vi "GetData.vi"() -> ()   [LabVIEW 2011]
uses:
  <vilib>/Platform/TimedLoop/XDataNode/timing_clust.ctl
  <vilib>/Platform/TimedLoop/XDataNode/nitl_modes.ctl
  <vilib>/Platform/TimedLoop/XDataNode/wakeup.ctl
  GlobalVariables.vi
  DS/DSRead int16.vi
  DS/DSRead uint8.vi
  DS/DSRead uint32.vi
  <vilib>/Platform/TimedLoop/XDataNode/XDataNode.xnode
  <vilib>/Platform/TimedLoop/XDataNode/XDNodeRunTimeDep.lvlib
  DS/DSWrite uint32.vi
panel:
  in  "Reinitialize?":bool
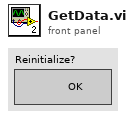
[diagram p1: front panel]
types:
  T1 = enum16{"Read", "Write", "ReadWrite", "BufferedRead", "BufferedReadWrite"}
  T2 = enum16{"OPC Server", "Global", "Dnet1", "Dnet2", "Dnet3", "Ain1", "Ain2", "Aout1", "Din1", "Din2", "Dout1"}
  T3 = typedef "XDNodeRunTimeDep.lvlib/timing_clust.ctl" = cluster{"Expected End [f-1]":u64, "Actual End [f-1]":u64, "Finished Late? [f-1]":bool, "Expected End [i-1]":u64, "Actual End [i-1]":u64, "Finished Late? [i-1]":bool, "Expected Start [i]":u64, "Actual Start [i]":u64, "Expected Start [f]":u64, "Actual Start [f]":u64, "Source Name":string, "Structure Name":string, "Period":i64, "Deadline":i64, "Offset":i64, "Start":i64, "Priority":i32, "Timeout":i32, "Mode":T4, "Wakeup Reason":T5, "Error":errorcluster, "Source Type":string, "Secondary Source Type":string, "Global End Time":u64, "Global Start Time":u64, "Frame Duration":u64, "Iteration Duration":u64, "Assigned CPU":i32, "I/O Scan Engine Mode":u32}
  T4 = typedef "XDNodeRunTimeDep.lvlib/nitl_modes.ctl" = enum32{"No Change", "Process missed periods, maintain original phase", "Discard missed periods, maintain original phase", "Process missed periods, ignore original phase", "Discard missed periods, ignore original phase"}
  T5 = typedef "XDNodeRunTimeDep.lvlib/wakeup.ctl" = enum32{"Normal", "Aborted", "Asynchronous wakeup", "Timing source error", "Timed loop error", "Timeout"}
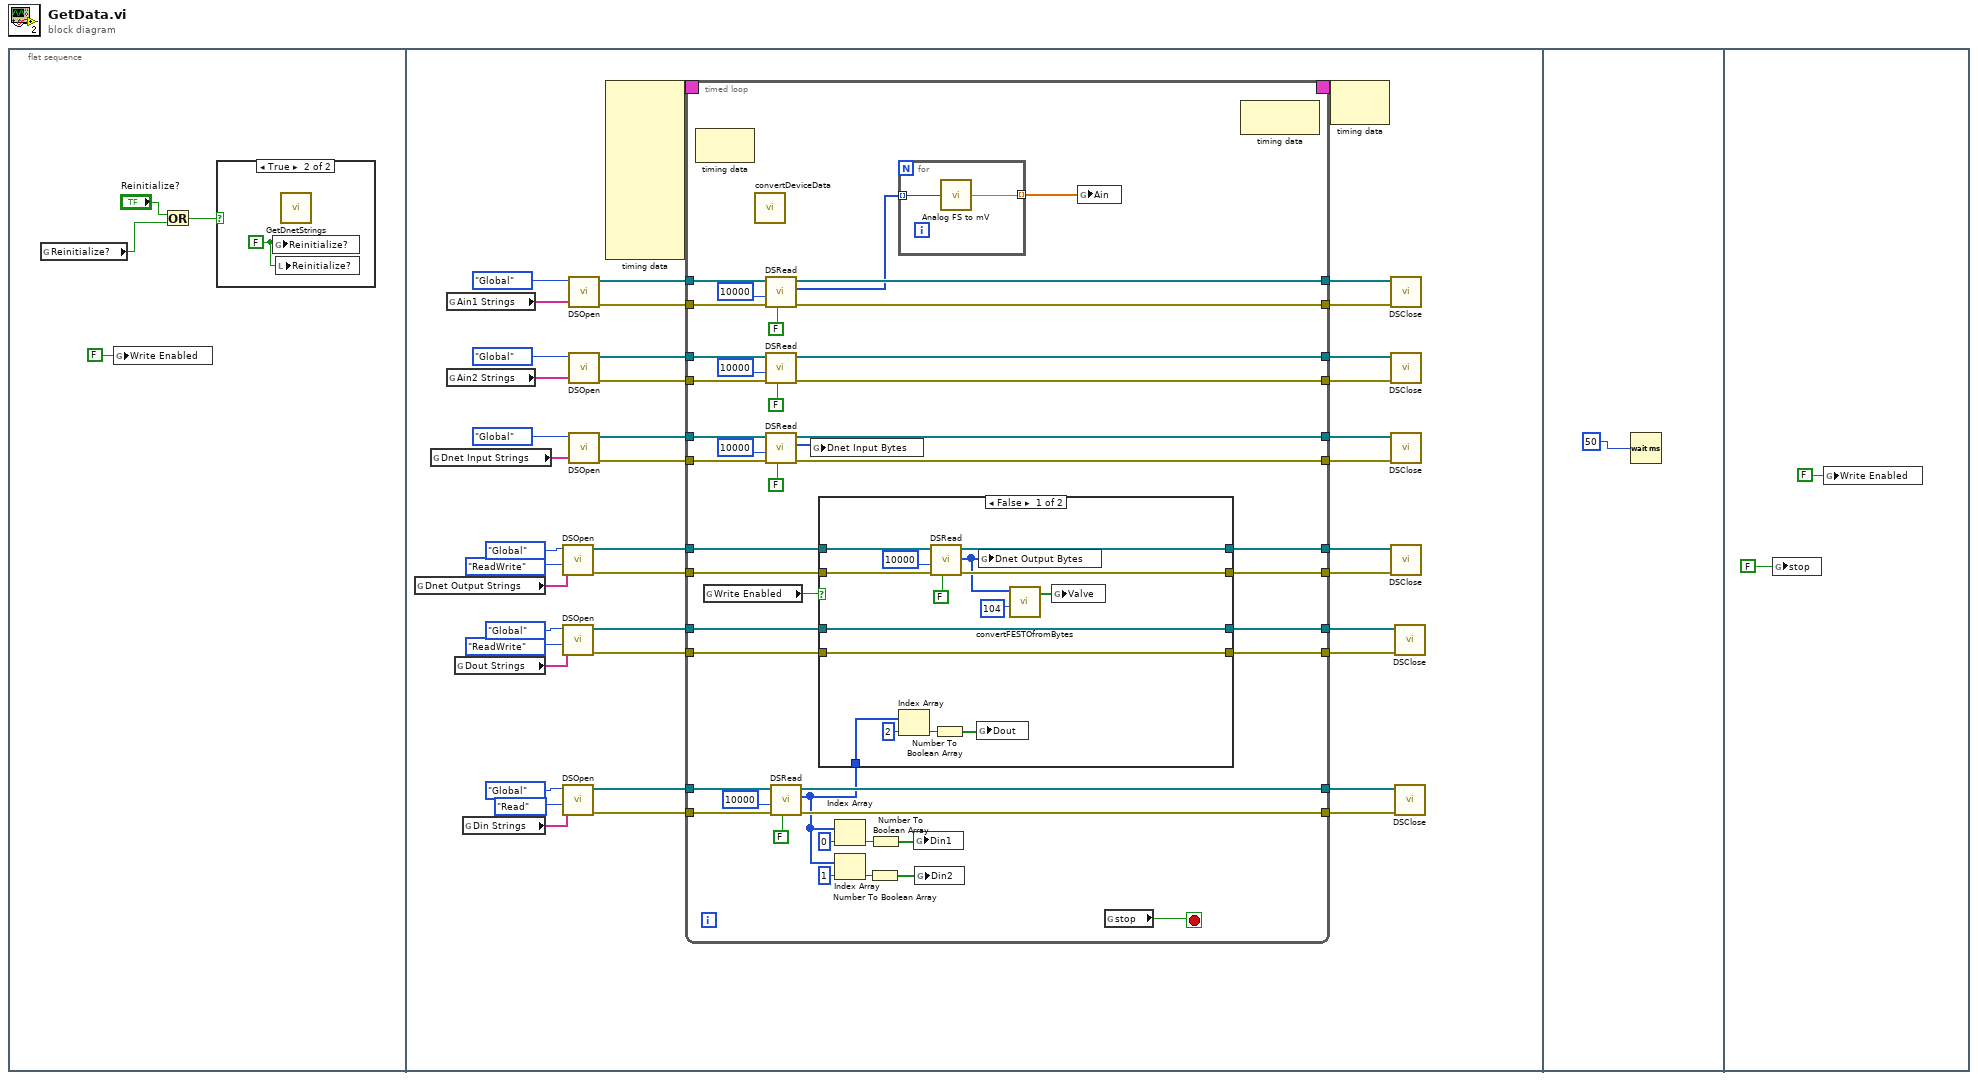
[diagram p0: block diagram]
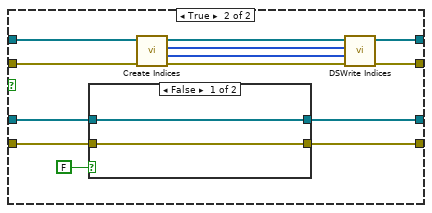
[diagram p3: hidden frame]
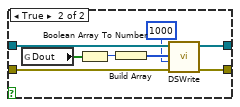
[diagram p4: hidden frame]
diagram:
  n1 = flat-sequence {
    frame #0 {
      n2 = global read "GlobalVariables.vi" "Reinitialize?"() -> (w3:bool)
      n3 = global write "GlobalVariables.vi" "Write Enabled"(FALSE ("Reinitialize?")) -> ()
      n4 = Or(x="Reinitialize?", y=w3) -> (x .or. y?=w2:bool)
      n5 = case shown="True" w2 {
        frame False {
        }
        frame True {
          w5 = FALSE
          n6 = global write "GlobalVariables.vi" "Reinitialize?"(w5) -> ()
          n7 = local write "Reinitialize?"(w5) -> ()
          n8 = call "GetDnetStrings.vi"() -> ()  [unwired: 12 in]
        }
      }
    }
    frame #1 {
      n9 = global read "GlobalVariables.vi" "Dnet Output Strings"() -> (w25:string[])
      n10 = global read "GlobalVariables.vi" "Dnet Input Strings"() -> (w31:string[])
      n11 = global read "GlobalVariables.vi" "Ain1 Strings"() -> (w43:string[])
      n12 = global read "GlobalVariables.vi" "Ain2 Strings"() -> (w37:string[])
      n13 = global read "GlobalVariables.vi" "Dout Strings"() -> (w11:string[])
      n14 = global read "GlobalVariables.vi" "Din Strings"() -> (w18:string[])
      n15 = call "DSOpen.vi"("Array"=w25, "mode"=T1."ReadWrite", "Slot"=T2."Global") -> ("error Out"=w23:errorcluster[], "connection out"=w22:refnum<k13>[])  [unwired: 7 in]
      n16 = call "DSOpen.vi"("Array"=w11, "mode"=T1."ReadWrite", "Slot"=T2."Global") -> ("error Out"=w9:errorcluster[], "connection out"=w8:refnum<k13>[])  [unwired: 7 in]
      n17 = call "DSOpen.vi"("Array"=w18, "mode"=T1."Read", "Slot"=T2."Global") -> ("error Out"=w16:errorcluster[], "connection out"=w15:refnum<k13>[])  [unwired: 7 in]
      n18 = call "DSOpen.vi"("Array"=w43, "Slot"=T2."Global") -> ("error Out"=w42:errorcluster[], "connection out"=w41:refnum<k13>[])  [unwired: 8 in]
      n19 = call "DSOpen.vi"("Array"=w37, "Slot"=T2."Global") -> ("error Out"=w36:errorcluster[], "connection out"=w35:refnum<k13>[])  [unwired: 8 in]
      n20 = call "DSOpen.vi"("Array"=w31, "Slot"=T2."Global") -> ("error Out"=w29:errorcluster[], "connection out"=w30:refnum<k13>[])  [unwired: 8 in]
      n21 = node-c288() -> (w46:T3)  [unwired: 10 in]
      n22 = timed-loop {
        tunnel: w42 -> [w89]
        tunnel: w41 -> [w88]
        tunnel: [w84] -> w40
        tunnel: [w83] -> w39
        tunnel: w36 -> [w79]
        tunnel: w35 -> [w78]
        tunnel: [w77] -> w34
        tunnel: [w76] -> w33
        tunnel: w30 -> [w73]
        tunnel: w29 -> [w72]
        tunnel: [w71] -> w27
        tunnel: [w70] -> w28
        timing: w46 -> [_]
        timing-out: [_] -> w45
        tunnel: w23 -> [w69]
        tunnel: w22 -> [w68]
        tunnel: [w67] -> w21
        tunnel: [w66] -> w20
        tunnel: w16 -> [w64]
        tunnel: w15 -> [w63]
        tunnel: [w54] -> w14
        tunnel: [w53] -> w13
        tunnel: w9 -> [w52]
        tunnel: w8 -> [w51]
        tunnel: [w50] -> w7
        tunnel: [w49] -> w6
        stop <- w90 stop-if-true
        n23 = node-c288() -> ()  [unwired: 1 in, 1 out]
        n24 = global read "GlobalVariables.vi" "Write Enabled"() -> (w65:bool)
        n25 = call "convertDeviceData.vi"() -> ()  [unwired: 12 in]
        n26 = call-poly "DSRead.vi"("wait for updated value (T)"=FALSE, "error in"=w89, "ms timeout (10000)"=10000, "connection in"=w88) -> ("error out"=w83:errorcluster[], "data"=w82:i16[], "connection out"=w84:refnum<k13>[])  [unwired: 5 in]
        n27 = call-poly "DSRead.vi"("wait for updated value (T)"=FALSE, "error in"=w79, "ms timeout (10000)"=10000, "connection in"=w78) -> ("error out"=w77:errorcluster[], "connection out"=w76:refnum<k13>[])  [unwired: 5 in, 1 out]
        n28 = call-poly "DSRead.vi"("wait for updated value (T)"=FALSE, "error in"=w72, "ms timeout (10000)"=10000, "connection in"=w73) -> ("error out"=w70:errorcluster[], "data"=w47:u8[], "connection out"=w71:refnum<k13>[])  [unwired: 5 in]
        n29 = call-poly "DSRead.vi"("wait for updated value (T)"=FALSE, "error in"=w64, "ms timeout (10000)"=10000, "connection in"=w63) -> ("error out"=w53:errorcluster[], "data"=w48:u32[], "connection out"=w54:refnum<k13>[])  [unwired: 5 in]
        n30 = global write "GlobalVariables.vi" "Dnet Input Bytes"(w47) -> ()
        n31 = case shown="False" w65 {
          tunnel: w69 -> [w103 w114]
          tunnel: w68 -> [w102 w113]
          tunnel: [w101 w111] -> w67
          tunnel: [w100 w112] -> w66
          tunnel: w52 -> [w98 w115]
          tunnel: w51 -> [w99 w116]
          tunnel: [w98 w118] -> w50
          tunnel: [w99 w117] -> w49
          tunnel: w48 -> [w95 _]
          frame False {
            n32 = Index Array(array=w95, index=2) -> (element=w91:u32)
            n33 = call-poly "DSRead.vi"("wait for updated value (T)"=FALSE, "error in"=w103, "ms timeout (10000)"=10000, "connection in"=w102) -> ("error out"=w101:errorcluster[], "data"=w94:u8[], "connection out"=w100:refnum<k13>[])  [unwired: 5 in]
            n34 = Number To Boolean Array(number=w91) -> (Boolean array=w96:bool[])
            n35 = global write "GlobalVariables.vi" "Dout"(w96) -> ()
            n36 = global write "GlobalVariables.vi" "Dnet Output Bytes"(w94) -> ()
            n37 = call "convertFESTOfromBytes.vi"("Start Byte"=104, "Bytes"=w94) -> ("data"=w92:bool[])  [unwired: 9 in]
            n38 = global write "GlobalVariables.vi" "Valve"(w92) -> ()
          }
          frame True {
            n39 = case shown="False" FALSE {
              tunnel: [w120 w128] -> w118
              tunnel: [w119 w127] -> w117
              tunnel: w116 -> [w119 w126]
              tunnel: w115 -> [w120 w125]
              frame False {
              }
              frame True {
                n40 = global read "GlobalVariables.vi" "Dout"() -> (w124:bool[])
                n41 = Boolean Array To Number(Boolean array=w124) -> (number=w123:u32)
                n42 = Build Array(w123) -> (w122:u32[])
                n43 = call-poly "DSWrite.vi"("error in"=w125, "ms timeout (10000)"=1000, "data"=w122, "connection in"=w126) -> ("error out"=w128:errorcluster[], "connection out"=w127:refnum<k13>[])  [unwired: 6 in]
              }
            }
            n44 = call "Create Indices.vi"("error in"=w114, "connection in"=w113) -> ("error out"=w110:errorcluster[], "Indices"=w108:i32[], "Dnet Output Bytes"=w106:u8[], "connection out"=w109:refnum<k13>[])  [unwired: 6 in]
            n45 = call "DSWrite Indices.vi"("error in"=w110, "Indices"=w108, "data"=w106, "connection in"=w109) -> ("error out"=w111:errorcluster[], "connection out"=w112:refnum<k13>[])  [unwired: 6 in]
          }
        }
        n46 = Index Array(array=w48, index=0) -> (element=w57:u32)
        n47 = Index Array(array=w48, index=1) -> (element=w58:u32)
        n48 = Number To Boolean Array(number=w58) -> (Boolean array=w56:bool[])
        n49 = Number To Boolean Array(number=w57) -> (Boolean array=w55:bool[])
        n50 = for {
          tunnel: w82 -> [w132] mode=indexing
          tunnel: [w131] -> w85 mode=indexing
          n51 = call "Analog FS to mV.vi"("input"=w132) -> ("output"=w131:dbl)
        }
        n52 = global write "GlobalVariables.vi" "Din1"(w55) -> ()
        n53 = global write "GlobalVariables.vi" "Din2"(w56) -> ()
        n54 = global write "GlobalVariables.vi" "Ain"(w85) -> ()
        n55 = global read "GlobalVariables.vi" "stop"() -> (w90:bool)
        n56 = node-c288() -> ()  [unwired: 1 in, 1 out]
      }
      n57 = node-c288(w45) -> ()  [unwired: 1 out]
      n58 = call "DSClose.vi"("error in (no error)"=w39, "connection id"=w40) -> ()  [unwired: 10 in]
      n59 = call "DSClose.vi"("error in (no error)"=w34, "connection id"=w33) -> ()  [unwired: 10 in]
      n60 = call "DSClose.vi"("error in (no error)"=w28, "connection id"=w27) -> ()  [unwired: 10 in]
      n61 = call "DSClose.vi"("error in (no error)"=w21, "connection id"=w20) -> ()  [unwired: 10 in]
      n62 = call "DSClose.vi"("error in (no error)"=w7, "connection id"=w6) -> ()  [unwired: 10 in]
      n63 = call "DSClose.vi"("error in (no error)"=w13, "connection id"=w14) -> ()  [unwired: 10 in]
    }
    frame #2 {
      n64 = Wait (ms)(milliseconds to wait=50) -> ()  [unwired: 1 out]
    }
    frame #3 {
      n65 = global write "GlobalVariables.vi" "stop"(FALSE ("stop")) -> ()
      n66 = global write "GlobalVariables.vi" "Write Enabled"(FALSE ("Reinitialize?")) -> ()
    }
  }
